vi "get display name.vi"(8 "error in":errorcluster, 11 "execution settings in":refnum<class "execution settings.lvclass">) -> (0 "error out":errorcluster, 2 "class name":string, 3 "execution settings out":refnum<class "execution settings.lvclass">)   [LabVIEW 2013, in "execution settings.lvclass"]
uses:
  execution settings.lvclass
  VI modification.lvclass
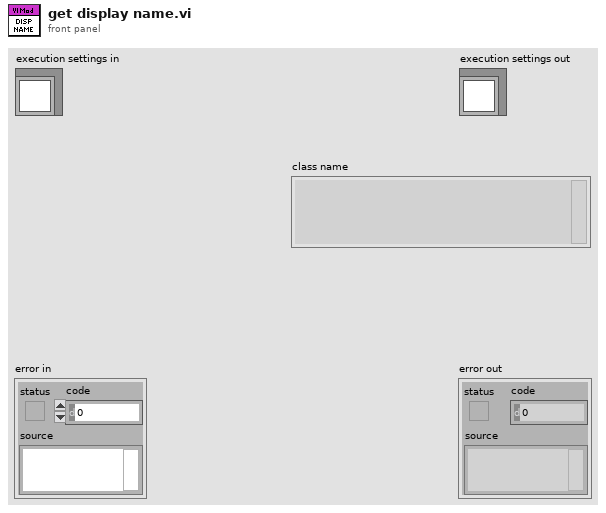
[diagram p1: front panel]
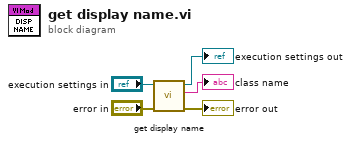
[diagram p0: block diagram]
diagram:
  n1 = call-parent "get display name.vi"("error in"="error in", "VI modification in"="execution settings in") -> ("error out"=→"error out":errorcluster, "class name"=→"class name":string, "VI modification out"=→"execution settings out":refnum<class "execution settings.lvclass">)  [unwired: 7 in]
